vi "_PC_Tab_CaptureData.vi"(7 "Function":enum16{"Init", "Get Data", "Update", "Close"}(ring), 8 "error in (no error)":errorcluster, 11 "tab ctrl refnums":T1) -> (0 "error out":errorcluster)   [LabVIEW 2018]
uses:
  RT/PublicSubVI/Ctl/_ctl_RT_D999_Param.ctl
  <vilib>/Utility/miscctls.llb/LVRowAndColumnTypeDef.ctl
  <vilib>/Utility/miscctls.llb/LVRowAndColumnUnsignedTypeDef.ctl
  PublicSubVI/Class/DataXML/DataXML dataType.ctl
  PublicSubVI/Class/DataXML/DataXML.lvclass
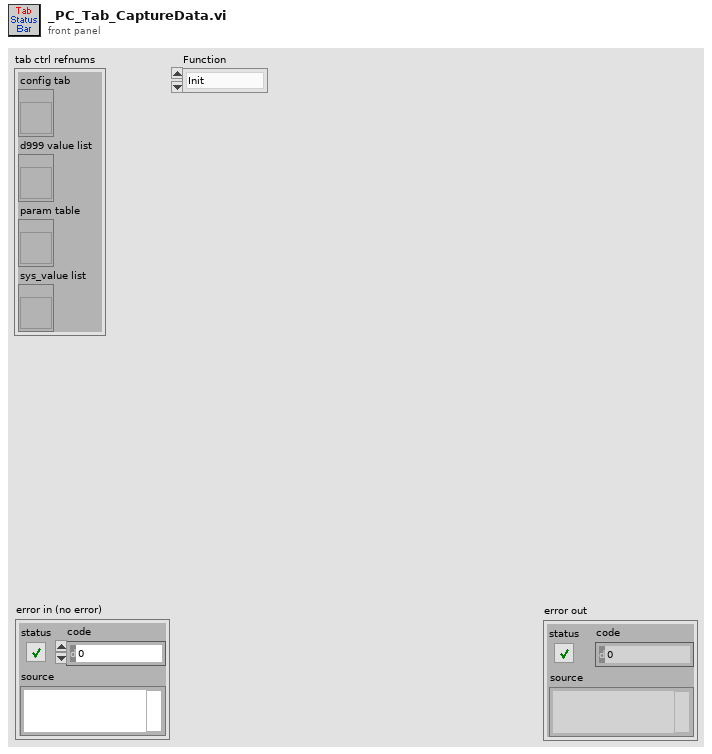
[diagram p1: front panel]
types:
  T1 = cluster{"config tab":refnum<vi>, "d999 value list":refnum<vi>, "param table":refnum<vi>, "sys_value list":refnum<vi>}
  T2 = typedef "LVRowAndColumnUnsignedTypeDef.ctl" = cluster{"Row":u32, "Column":u32}
  T3 = typedef "LVRowAndColumnTypeDef.ctl" = cluster{"Row":i32, "Column":i32}
  T4 = typedef "DataXML dataType.ctl" = enum16{"Instrument", "UserInterface", "SampleType", "UserDefined"}
  T5 = typedef "_ctl_RT_D999_Param.ctl" = cluster{"Enable":bool, "AI":cluster{"Label":string, "MultiValue":dbl, "AddValue":dbl}[], "AO":i16[], "Switch":bool[]}
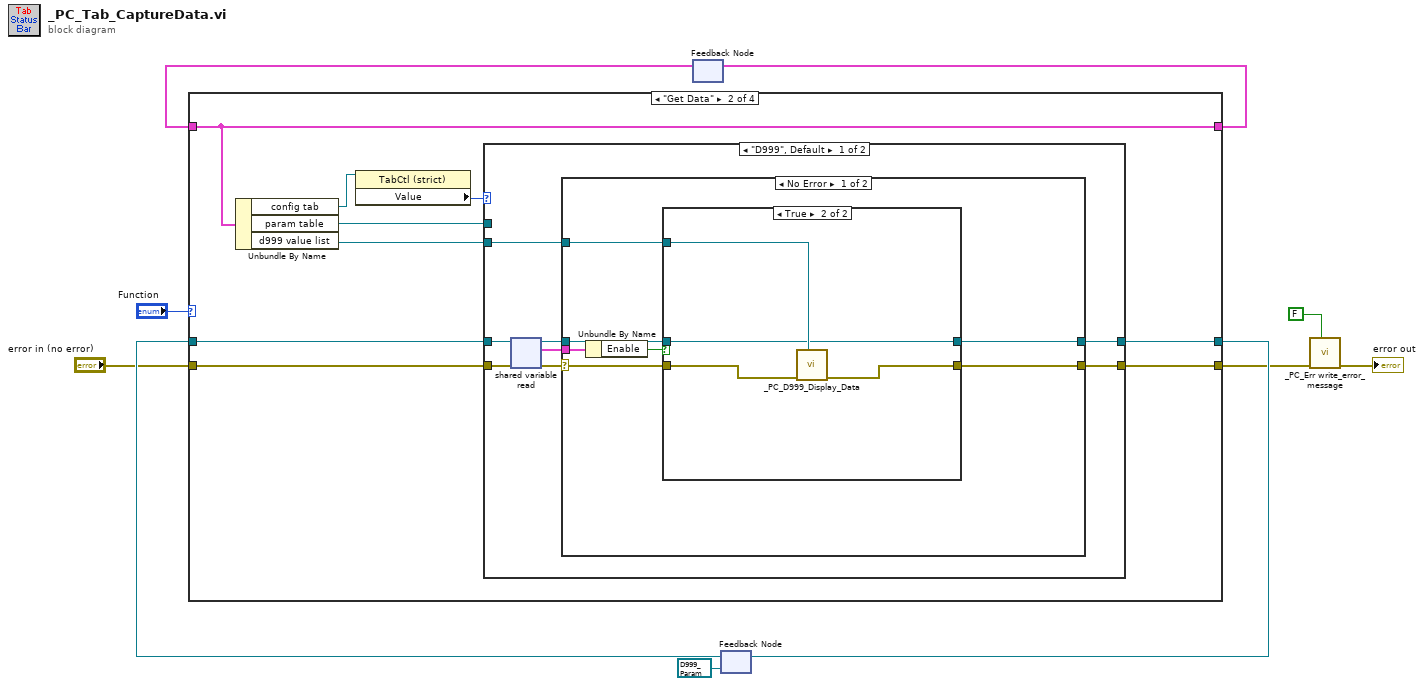
[diagram p0: block diagram]
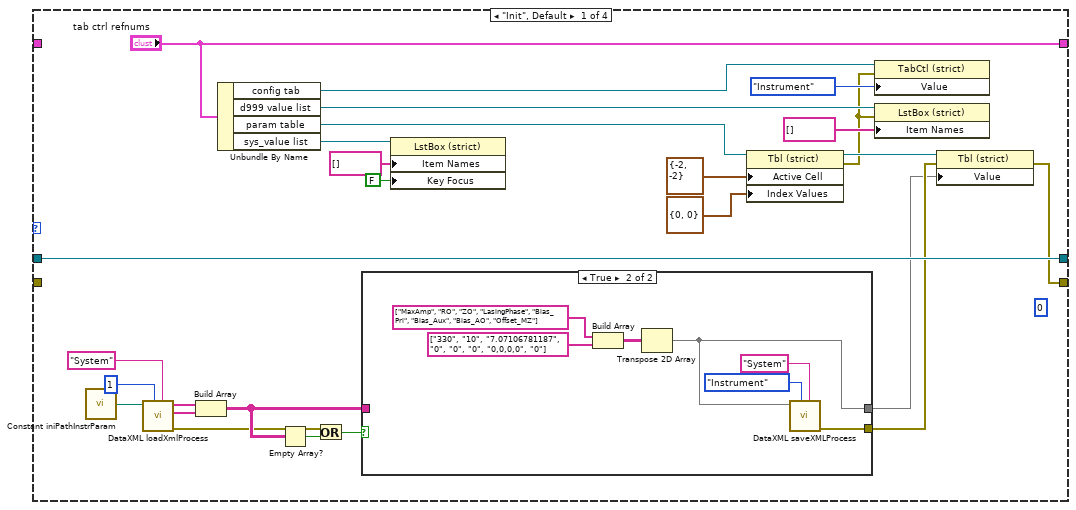
[diagram p2: hidden frame]
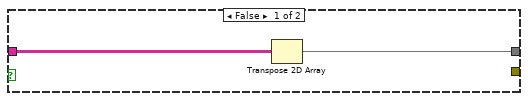
[diagram p3: hidden frame]
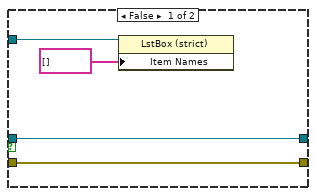
[diagram p4: hidden frame]
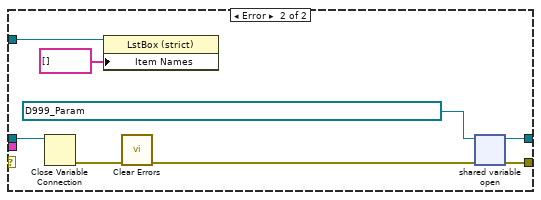
[diagram p5: hidden frame]
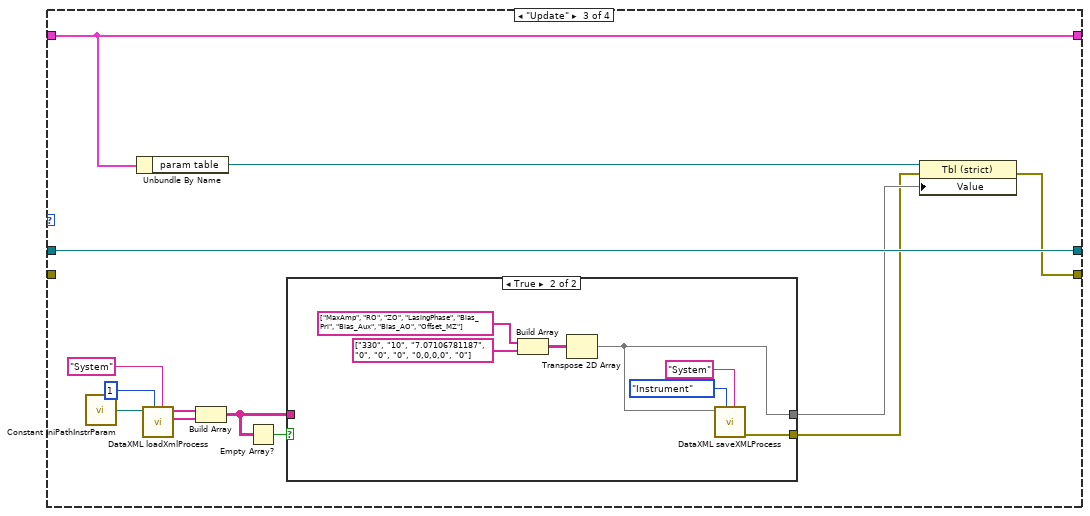
[diagram p7: hidden frame]
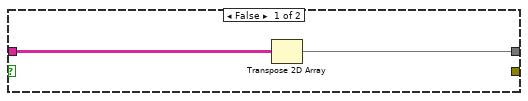
[diagram p8: hidden frame]
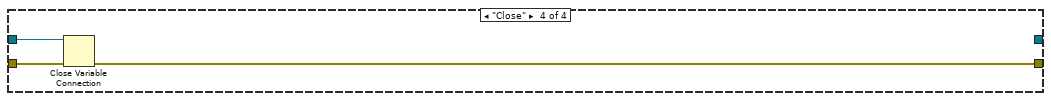
[diagram p9: hidden frame]
diagram:
  n1 = feedback #1() -> (w8:T1)  [unwired: 1 in]
  n2 = feedback #2(refnum<k21> refnum ("shared variable refnum in")) -> (w6:refnum<k21>)
  n3 = case shown="\"Get Data\"" "Function" {
    tunnel: ["tab ctrl refnums" w54 w92 _] -> w9
    tunnel: w8 -> [_ w54 w92 _]
    tunnel: w6 -> [w34 w49 w95 w112]
    tunnel: [w34 w48 w95 _] -> w7
    tunnel: [w20 w47 w93 w110] -> w3
    tunnel: "error in (no error)" -> [_ w46 _ w111]
    frame "Init", Default {
      (unwired) u8 0 ("f")
      n4 = call "Constant iniPathInstrParam.vi"() -> ("appended path"=w26:path)
      n5 = call "DataXML loadXmlProcess.vi"("target name"="System", "level"=u8 1, "xml_data_path"=w26) -> ("error IO"=w13:errorcluster, "value"=w23:string[], "name"=w24:string[])  [unwired: 5 in, 1 out]
      n6 = Build Array(w24, w23) -> (w14:string[][])
      n7 = Unbundle By Name("tab ctrl refnums") -> ("config tab"=w36:refnum<vi>, "d999 value list"=w31:refnum<vi>, "param table"=w30:refnum<vi>, "sys_value list"=w18:refnum<vi>)
      n8 = Empty Array?(array=w14) -> (empty?=w12:bool)
      n9 = Or(x=w13, y=w12) -> (x .or. y?=w11:bool)
      n10 = case shown="True" w11 {
        tunnel: w14 -> [w38 _]
        tunnel: [_ w43] -> w21
        tunnel: [w37 w39] -> w15
        frame False {
          n11 = Transpose 2D Array(2D array=w38) -> (transposed array=w37:string[][])
        }
        frame True {
          n12 = Build Array(string[] ["MaxAmp", "RO", "ZO", "LasingPhase", "Bias_Pri", "Bias_Aux", "Bias_AO", "Offset_MZ"], string[] ["330", "10", "7.07106781187", "0", "0", "0", "0,0,0,0", "0"]) -> (w40:string[][])
          n13 = Transpose 2D Array(2D array=w40) -> (transposed array=w39:string[][])
          n14 = call "DataXML saveXMLProcess.vi"("addTagName"="System", "dataType"=DataXML_dataType."Instrument", "newData"=w39) -> ("error out"=w43:errorcluster)  [unwired: 8 in]
        }
      }
      n15 = property class="LstBox (strict)"(reference=w18, "Item Names"=string[] [], "Key Focus"=FALSE) -> ()  [unwired: 1 in, 2 out]
      n16 = property class="Tbl (strict)"(reference=w30, "Active Cell"=T3 {"Row"=-2, "Column"=-2} ("Active Cell:Active Cell"), "Index Values"=T2 {"Row"=0, "Column"=0}) -> (reference out=w29:refnum<vi>, error out=w27:errorcluster)  [unwired: 1 in]
      n17 = property class="TabCtl (strict)"(reference=w36, error in=w27, "Value"=enum32{"D999", "Instrument"}."Instrument") -> ()  [unwired: 2 out]
      n18 = property class="LstBox (strict)"(reference=w31, error in=w27, "Item Names"=string[] []) -> ()  [unwired: 2 out]
      n19 = property class="Tbl (strict)"(reference=w29, error in=w21, "Value"=w15) -> (error out=w20:errorcluster)  [unwired: 1 out]
    }
    frame "Get Data" {
      n20 = Unbundle By Name(w54) -> ("config tab"=w53:refnum<vi>, "param table"=w50:refnum<vi>, "d999 value list"=w51:refnum<vi>)
      n21 = property class="TabCtl (strict)"(reference=w53) -> ("Value"=w52:enum32{"D999", "Instrument"})  [unwired: 1 in, 2 out]
      n22 = case shown="\"D999\", Default" w52 {
        tunnel: w51 -> [w62 _]
        tunnel: w49 -> [w61 w87]
        tunnel: [w57 w87] -> w48
        tunnel: w50 -> [_ _]
        tunnel: [w56 w86] -> w47
        tunnel: w46 -> [w55 w86]
        frame "D999", Default {
          n23 = shared-variable-read(w61, w55) -> (w58:refnum<k21>, w59:errorcluster, w60:T5)
          n24 = case shown="No Error" w59 {
            selector: w59 -> [w68 _]
            tunnel: w62 -> [w69 w85]
            tunnel: w60 -> [w67 _]
            tunnel: w58 -> [w64 w83]
            tunnel: [w65 w81] -> w57
            tunnel: [w63 w78] -> w56
            frame No Error {
              n25 = Unbundle By Name(w67) -> ("Enable"=w66:bool)
              n26 = case shown="True" w66 {
                tunnel: w69 -> [w72 w77]
                tunnel: w68 -> [w70 w76]
                tunnel: [w71 w75] -> w65
                tunnel: w64 -> [w71 w75]
                tunnel: [w70 w74] -> w63
                frame False {
                  n27 = property on="Property Node" class="LstBox (strict)"(reference=w72, "Item Names"=string[] []) -> ()  [unwired: 1 in, 2 out]
                }
                frame True {
                  n28 = call "_PC_D999_Display_Data.vi"("Listbox"=w77, "error in"=w76) -> ("error out"=w74:errorcluster)  [unwired: 9 in]
                }
              }
            }
            frame Error {
              n29 = Close Variable Connection(11:w83) -> (0:w80:errorcluster)  [unwired: 1 in]
              n30 = property on="Property Node" class="LstBox (strict)"(reference=w85, "Item Names"=string[] []) -> ()  [unwired: 1 in, 2 out]
              n31 = call <vilib>:"Clear Errors.vi"("error in (no error)"=w80) -> ("error out"=w79:errorcluster)  [unwired: 5 in, 1 out]
              n32 = shared-variable-open(refnum<k21> "ni.var.psp://NI-sbRIO/_RT_CtrlLoop_D999_Variables/D999_UserParam" ("shared variable refnum in"), w79) -> (w81:refnum<k21>, w78:errorcluster)
            }
          }
        }
        frame "Instrument" {
        }
      }
    }
    frame "Update" {
      n33 = call "Constant iniPathInstrParam.vi"() -> ("appended path"=w100:path)
      n34 = Unbundle By Name(w92) -> ("param table"=w94:refnum<vi>)
      n35 = call "DataXML loadXmlProcess.vi"("target name"="System", "level"=u8 1, "xml_data_path"=w100) -> ("value"=w97:string[], "name"=w98:string[])  [unwired: 5 in, 2 out]
      n36 = Build Array(w98, w97) -> (w89:string[][])
      n37 = Empty Array?(array=w89) -> (empty?=w88:bool)
      n38 = case shown="True" w88 {
        tunnel: w89 -> [w102 _]
        tunnel: [_ w107] -> w90
        tunnel: [w101 w103] -> w91
        frame False {
          n39 = Transpose 2D Array(2D array=w102) -> (transposed array=w101:string[][])
        }
        frame True {
          n40 = Build Array(string[] ["MaxAmp", "RO", "ZO", "LasingPhase", "Bias_Pri", "Bias_Aux", "Bias_AO", "Offset_MZ"], string[] ["330", "10", "7.07106781187", "0", "0", "0", "0,0,0,0", "0"]) -> (w104:string[][])
          n41 = Transpose 2D Array(2D array=w104) -> (transposed array=w103:string[][])
          n42 = call "DataXML saveXMLProcess.vi"("addTagName"="System", "dataType"=DataXML_dataType."Instrument", "newData"=w103) -> ("error out"=w107:errorcluster)  [unwired: 8 in]
        }
      }
      n43 = property class="Tbl (strict)"(reference=w94, error in=w90, "Value"=w91) -> (error out=w93:errorcluster)  [unwired: 1 out]
    }
    frame "Close" {
      n44 = Close Variable Connection(8:w111, 11:w112) -> (0:w110:errorcluster)
    }
  }
  n45 = feedback-in #1(w9) -> ()
  n46 = feedback-in #2(w7) -> ()
  n47 = call "_PC_Err write_error_message.vi"("show msg( T )"=FALSE, "error in"=w3) -> ("error out"=→"error out":errorcluster)  [unwired: 9 in]
